vi "Configure Offset.vi"(5 "Phase Offset Unit (0: Degrees)":i32(ring) items=["Degrees", "Radians"], 6 "Phase Offset (0)":dbl, 7 "Magnitude Offset Slope (0 dB/GHz)":dbl, 8 "error in (no error)":errorcluster, 9 "Magnitude Offset (0 dB)":dbl, 10 "Channel (1)":i32=1, 11 "VISA resource name":refnum<visa-resource-name>) -> (0 "error out":errorcluster, 3 "VISA resource name out":refnum<visa-resource-name>)   [LabVIEW 2018, in "Keysight PNA Series.lvlib"]
doc: "Configures the offest of the data trace magnitude and phase."
uses:
  Keysight PNA Series.lvlib
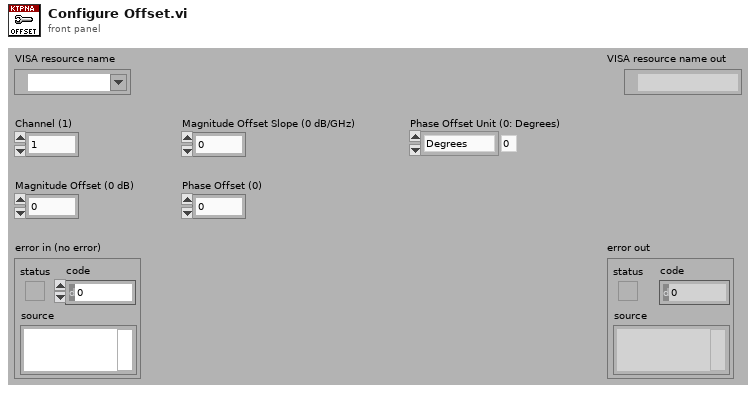
[diagram p1: front panel]
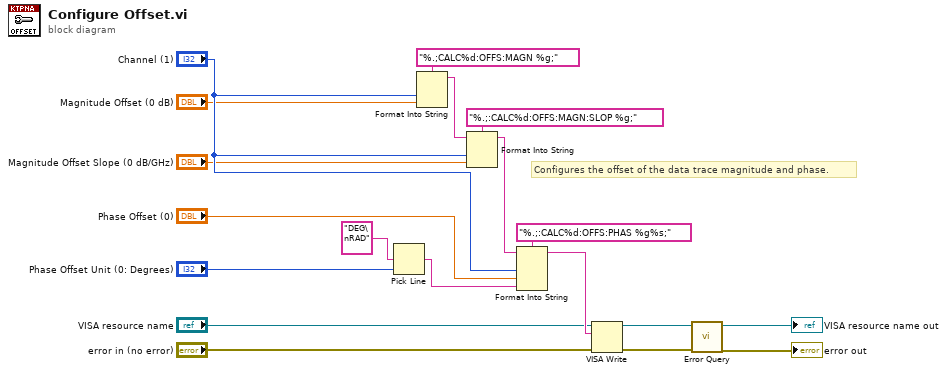
[diagram p0: block diagram]
diagram:
  # "Configures the offset of the data trace magnitude and phase."
  n1 = Pick Line(multi-line string="DEG\nRAD", line index="Phase Offset Unit (0: Degrees)") -> (output string=w8:string)  [unwired: 1 in]
  n2 = Format Into String(format string="%.;CALC%d:OFFS:MAGN %g;", "Channel (1)", "Magnitude Offset (0 dB)") -> (resulting string=w16:string)  [unwired: 2 in, 1 out]
  n3 = Format Into String(format string="%.;:CALC%d:OFFS:MAGN:SLOP %g;", initial string=w16, "Channel (1)", "Magnitude Offset Slope (0 dB/GHz)") -> (resulting string=w11:string)  [unwired: 1 in, 1 out]
  n4 = Format Into String(format string="%.;:CALC%d:OFFS:PHAS %g%s;", initial string=w11, "Channel (1)", "Phase Offset (0)", w8) -> (resulting string=w7:string)  [unwired: 1 in, 1 out]
  n5 = VISA Write(VISA resource name="VISA resource name", write buffer=w7, error in (no error)="error in (no error)") -> (VISA resource name out=w4:refnum<visa-resource-name>, error out=w3:errorcluster)  [unwired: 1 out]
  n6 = call "Error Query.vi"("error in (no error)"=w3, "VISA resource name"=w4) -> ("error out"=→"error out":errorcluster, "VISA resource name out"=→"VISA resource name out":refnum<visa-resource-name>)  [unwired: 6 in, 2 out]
